vi "3.3 - Lidar DS Slicer.vi"(3 "Low Slice":dbl, 4 "Numer of Cells to be low":dbl, 5 "High Slice":dbl, 6 "Numer of Cells to be high":dbl) -> (0 "Low lower bound":dbl, 1 "Low upper bound":dbl, 2 "Total iterations":dbl)   [LabVIEW 2010]
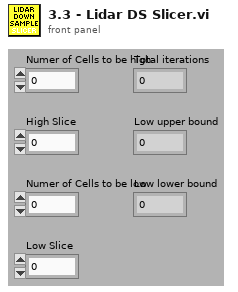
[diagram p1: front panel]
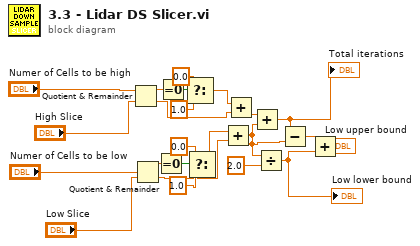
[diagram p0: block diagram]
diagram:
  n1 = Quotient & Remainder(x="Numer of Cells to be high", y="High Slice") -> (x-y*floor(x/y)=w3:dbl, floor(x/y)=w10:dbl)
  n2 = Quotient & Remainder(x="Numer of Cells to be low", y="Low Slice") -> (x-y*floor(x/y)=w8:dbl, floor(x/y)=w11:dbl)
  n3 = Equal To 0?(x=w8) -> (x = 0?=w22:bool)
  n4 = Equal To 0?(x=w3) -> (x = 0?=w4:bool)
  n5 = Select(t=0.0, s=w4, f=1.0) -> (s? t:f=w9:dbl)
  n6 = Select(t=0.0, s=w22, f=1.0) -> (s? t:f=w12:dbl)
  n7 = Add(x=w12, y=w11) -> (x+y=w16:dbl)
  n8 = Add(x=w9, y=w10) -> (x+y=w13:dbl)
  n9 = Add(x=w13, y=w16) -> (x+y=w15:dbl)
  "Total iterations" <- w15
  n10 = Divide(x=w16, y=2.0) -> (x/y=w17:dbl)
  "Low lower bound" <- w17
  n11 = Subtract(x=w15, y=w16) -> (x-y=w18:dbl)
  n12 = Add(x=w18, y=w17) -> (x+y=→"Low upper bound":dbl)
